vi "Begin(not).vi"(8 "error in":errorcluster) -> (0 "error out":errorcluster)   [LabVIEW 2016]
doc: "Called before other user functions, this VI is expected to open initial I/O refnums, load in file data, and do all program initialization. Notice that the <B>error out</B> terminal is simply used for data flow. Wiring it to other structures or subVIs ensures that this VI runs first."
uses:
  <vilib>/Rock Robotics/WPI/DriverStation/WPI_DriverStationRobotMode2.ctl
  <vilib>/Rock Robotics/WPI/Joystick/WPI_JoystickDeviceEnum.ctl
  <vilib>/Rock Robotics/WPI/ThirdParty/CanMotor/TalonSRX/WPI_CANTalonSRX_APIControlMode.ctl
  <vilib>/Rock Robotics/WPI/ThirdParty/CanMotor/TalonSRX/WPI_CANTalonSRX_APIFeedbackSelect.ctl
  <vilib>/Rock Robotics/SystemInterfaces/DIO/FPGA_DIOChannel.ctl
  <vilib>/Rock Robotics/SystemInterfaces/DIO/FPGA_DIOPWMChannel.ctl
  <vilib>/Rock Robotics/WPI/SafetyOutput/WPI_SafetyOutputConfigMenu.ctl
  Robot Global Data.vi
  <vilib>/Rock Robotics/Network Tables/NT Write String Array.vi
  <vilib>/Rock Robotics/WPI/Counter/WPI_CounterDigitalInputToDigitalSource.vi
  <vilib>/Rock Robotics/WPI/Switch/WPI_SwitchOpenLimit.vi
  <vilib>/Rock Robotics/WPI/RobotDrive/WPI_RobotDriveOpen4MotorWithExistingMotors.vi
  <vilib>/Rock Robotics/WPI/RobotDrive/WPI_RobotDriveOpen4MotorWithTalon.vi
  <vilib>/Rock Robotics/WPI/MotorControl/WPI_MotorControlOpen SPARK.vi
  <vilib>/Rock Robotics/WPI/MotorControl/WPI_MotorControlOpen Victor.vi
  <vilib>/Rock Robotics/WPI/Solenoid/WPI_SolenoidOpenSingle.vi
  <vilib>/Rock Robotics/WPI/Solenoid/WPI_SolenoidChannel.ctl
panel:
  in  "Number Encoder Lines\n(Counts Per Rotation)":u32=309
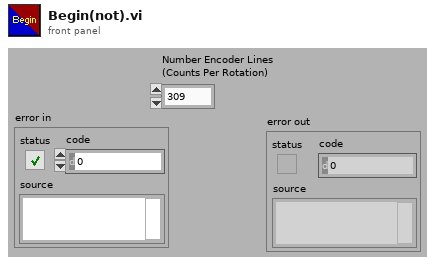
[diagram p1: front panel]
types:
  T1 = typedef "FPGA_DIOChannel.ctl" = enum8{"DIO 0", "DIO 1", "DIO 2", "DIO 3", "DIO 4", "DIO 5", "DIO 6", "DIO 7", "DIO 8", "DIO 9", "DIO MXP 0", "DIO MXP 1", "DIO MXP 2", "DIO MXP 3", "DIO MXP 4", "DIO MXP 5", "DIO MXP 6", "DIO MXP 7", "DIO MXP 8", "DIO MXP 9", "DIO MXP 10", "DIO MXP 11", "DIO MXP 12", "DIO MXP 13", "DIO MXP 14", "DIO MXP 15", "SPI Port CS1", "SPI Port CS2", "SPI Port CS3", "SPI Port MISO", "SPI Port MOSI", "Invalid"}
  T2 = typedef "WPI_CANTalonSRX_APIFeedbackSelect.ctl" = enum16{"Digital Quadrature Encoder", "Analog Potentiometer", "Analog Encoder", "Count on Quad-A (Rising-Edge)", "Count on Quad-A (Falling-Edge)", "CTR Magnetic Enc (Absolute)", "CTR Magnetic Enc (Relative)", "Pulse Width"}
  T3 = typedef "WPI_CANTalonSRX_APIControlMode.ctl" = enum8{"Percent VBus", "Speed", "Position", "Slave", "Unchanged / Invalid", "Voltage Compensation", "Current", "Motion Profile", "Motion Magic"}
  T4 = typedef "WPI_JoystickDeviceEnum.ctl" = enum16{"USB 0", "USB 1", "USB 2", "USB 3", "USB 4", "USB 5"}
  T5 = typedef "WPI_DriverStationRobotMode2.ctl" = enum16{"Autonomous Disabled", "Autonomous Enabled", "Teleop Disabled", "Teleop Enabled", "Disconnected", "Finish", "Test Disabled", "Test Enabled", "Emergency Stopped"}
  T6 = typedef "WPI_MotorControlDeviceRef.ctl" = cluster{"DeviceStatus":errorcluster, "Type":T7, "PWM":cluster{"PWM Channel":T8, "DeadBand":T9}, "CAN":cluster{"Device Number":u8, "SetOutput VI Ref":variant, "GetOutput VI Ref":variant, "Enable VI Ref":variant, "Disable VI Ref":variant, "Data":variant}, "Invert":bool}
  T7 = typedef "WPI_MotorControlType.ctl" = enum16{"PWM", "CAN"}
  T8 = typedef "FPGA_DIOPWMChannel.ctl" = enum8{"PWM 0", "PWM 1", "PWM 2", "PWM 3", "PWM 4", "PWM 5", "PWM 6", "PWM 7", "PWM 8", "PWM 9", "PWM MXP 0", "PWM MXP 1", "PWM MXP 2", "PWM MXP 3", "PWM MXP 4", "PWM MXP 5", "PWM MXP 6", "PWM MXP 7", "PWM MXP 8", "PWM MXP 9", "Invalid"}
  T9 = typedef "WPI_PWMDeadband.ctl" = cluster{"Name":string, "maxPositivePwm":i32, "minPositivePwm":i32, "centerPwm":i32, "maxNegativePwm":i32, "minNegativePwm":i32, "angularRange":u16}
  T10 = typedef "WPI_SafetyOutputConfigMenu.ctl" = enum16{"Enable", "Disable"}
  T11 = typedef "WPI_RobotDriveDevRef.ctl" = cluster{"DevStatus":errorcluster, "Motors[]":T6[], "Square Inputs":bool, "Max Output":dbl}
  T12 = typedef "WPI_ServoDeviceRef.ctl" = cluster{"DeviceStatus":errorcluster, "PWM Channel":T8, "DeadBand":T9}
  T13 = typedef "WPI_JoystickDevRef.ctl" = cluster{"Device":T4}
  T14 = typedef "WPI_SwitchDevRef.ctl" = cluster{"DevStatus":errorcluster, "DIO Channel":T1, "CntIndex":T15, "Normally Closed":bool}
  T15 = typedef "FPGA_CounterCtrSystemIndex.ctl" = enum8{"Ctr 0", "Ctr 1", "Ctr 2", "Ctr 3", "Ctr 4", "Ctr 5", "Ctr 6", "Ctr 7", "Invalid"}
  T16 = typedef "WPI_SolenoidChannel.ctl" = enum8{"Solenoid 0", "Solenoid 1", "Solenoid 2", "Solenoid 3", "Solenoid 4", "Solenoid 5", "Solenoid 6", "Solenoid 7", "Invalid"}
  T17 = typedef "WPI_SolenoidDevRef.ctl" = cluster{"DevStatus":errorcluster, "Pneumatics Control Module":u8, "Forward Solenoid Channel":T16, "Reverse Solenoid Channel":T16}
  T18 = typedef "WPI_DigitalInputDevRef.ctl" = cluster{"DevStatus":errorcluster, "DIO Channel":T1}
  T19 = typedef "FPGA_CounterEncoderSourceConvertionLVSourceType.ctl" = cluster{"DevStatus":errorcluster, "AnalogTriggerMode?":bool, "DigitalMode":cluster{"DIO Channel":T20}, "AnalogTriggerMode":cluster{"AnalogTriggerIndex":T21, "OutputType":T22}}
  T20 = typedef "FPGA_DIODigitalSourceChannel.ctl" = enum8{"DIO 0", "DIO 1", "DIO 2", "DIO 3", "DIO 4", "DIO 5", "DIO 6", "DIO 7", "DIO 8", "DIO 9", "DIO MXP 0", "DIO MXP 1", "DIO MXP 2", "DIO MXP 3", "DIO MXP 4", "DIO MXP 5", "DIO MXP 6", "DIO MXP 7", "DIO MXP 8", "DIO MXP 9", "DIO MXP 10", "DIO MXP 11", "DIO MXP 12", "DIO MXP 13", "DIO MXP 14", "DIO MXP 15", "Disabled"}
  T21 = typedef "FPGA_AnalogTriggerIndex.ctl" = enum8{"Trig 0", "Trig 1", "Trig 2", "Trig 3", "Trig 4", "Trig 5", "Trig 6", "Trig 7", "Invalid"}
  T22 = typedef "FPGA_AnalogTriggerOutType.ctl" = enum16{"InWindow", "TriggerState", "Rising", "Falling"}
  T23 = typedef "WPI_EncoderDevRef.ctl" = cluster{"DevStatus":errorcluster, "EncoderIndex":T24, "CounterIndex":T15, "DistancePerCount":dbl, "Decoding Type":T25}
  T24 = typedef "FPGA_EncoderIdx.ctl" = enum8{"Enc 0", "Enc 1", "Enc 2", "Enc 3", "Enc 4", "Enc 5", "Enc 6", "Enc 7", "Invalid"}
  T25 = typedef "WPI_EncoderType.ctl" = enum16{"1x", "2x", "4x"}
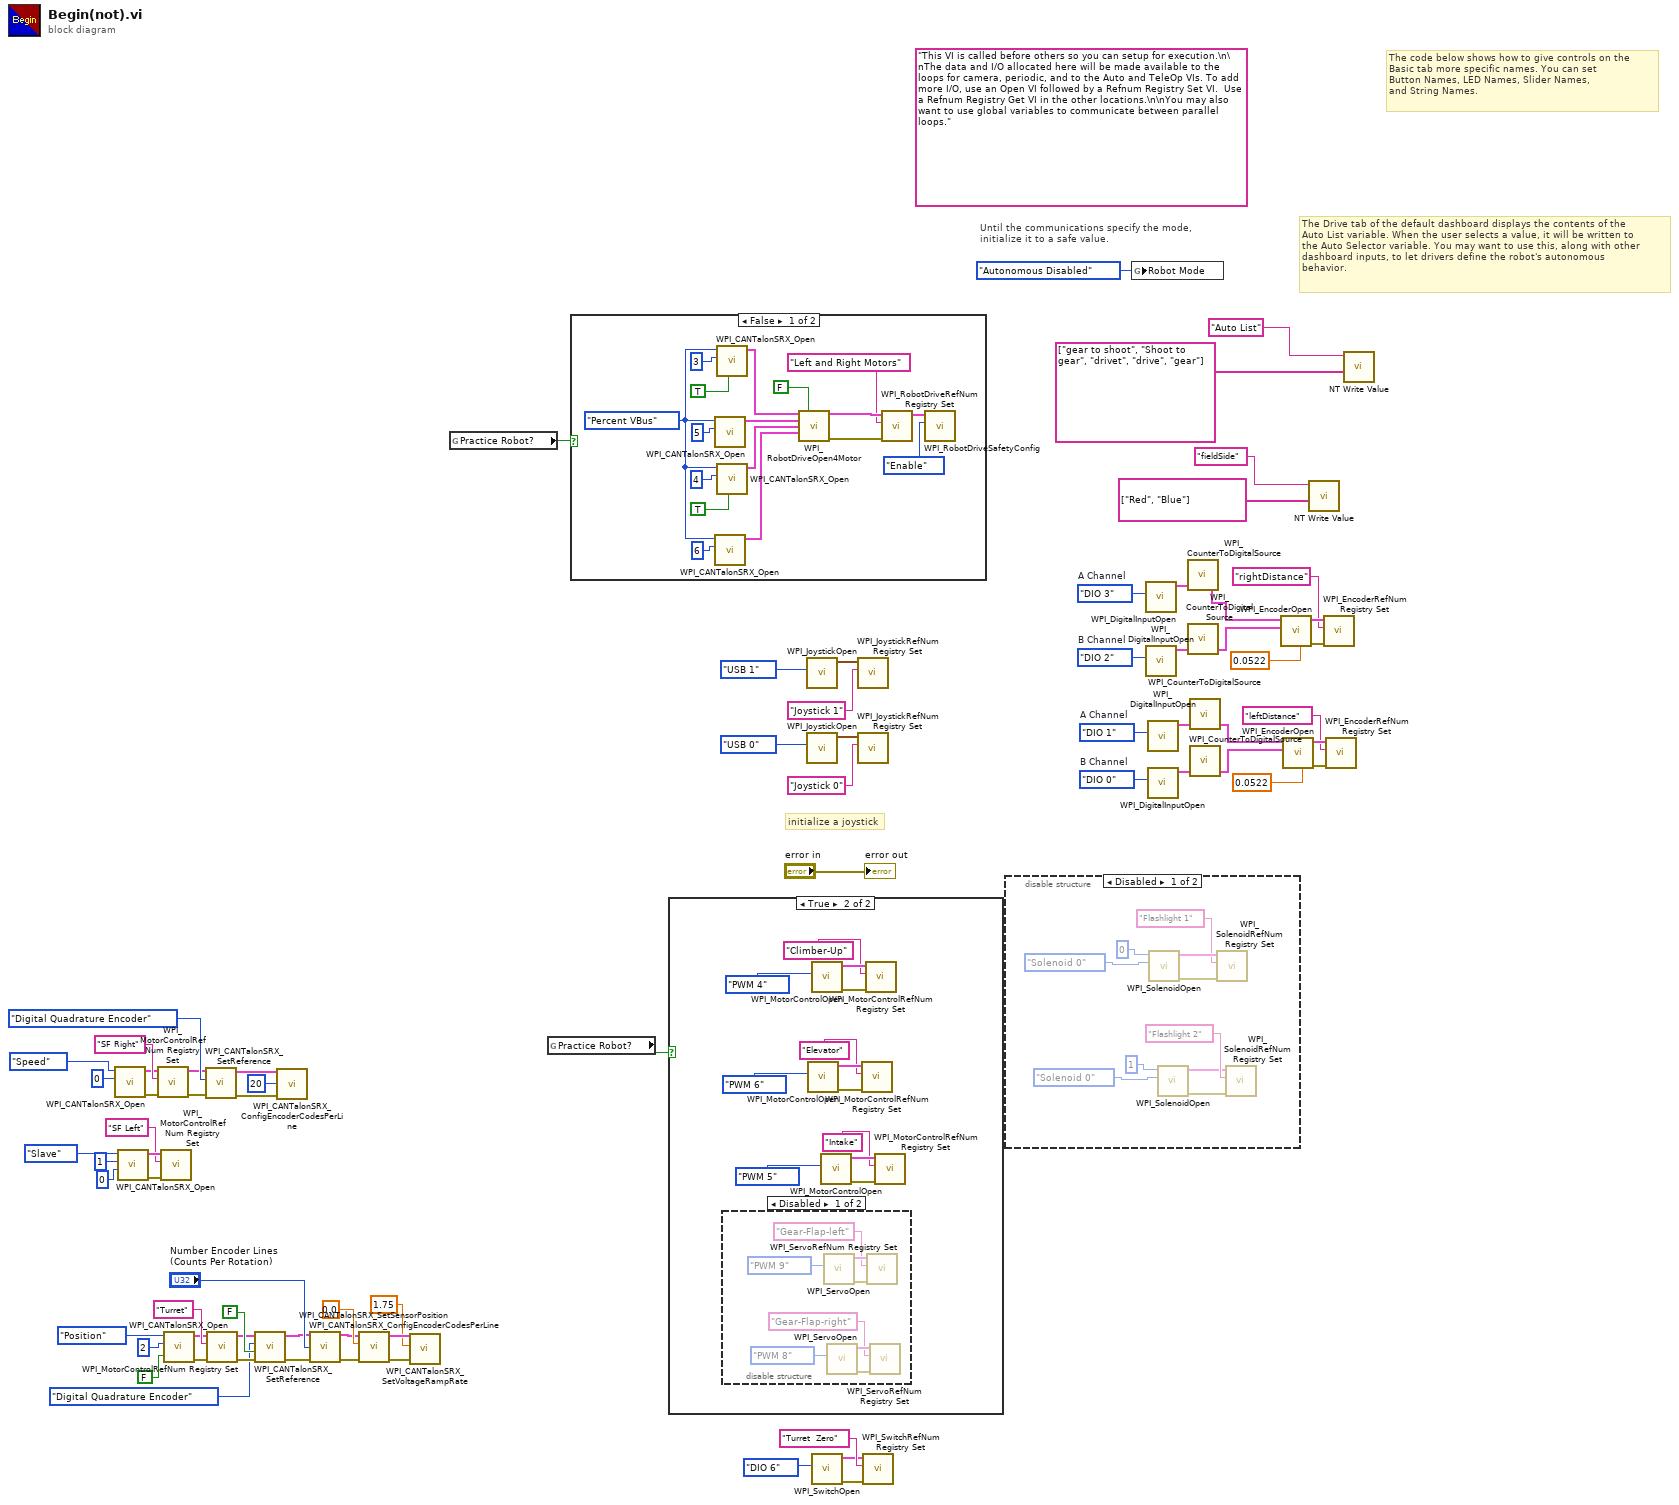
[diagram p0: block diagram]
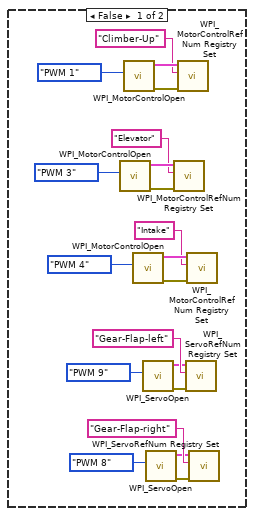
[diagram p3: hidden frame]
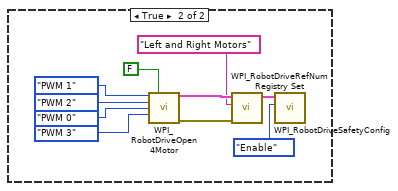
[diagram p5: hidden frame]
diagram:
  w18 = FPGA_DIOChannel."DIO 2"  # B Channel
  w17 = FPGA_DIOChannel."DIO 3"  # A Channel
  w27 = FPGA_DIOChannel."DIO 0"  # B Channel
  w26 = FPGA_DIOChannel."DIO 1"  # A Channel
  (unwired) "This VI is called before others so you can setup for execution.\n\nThe data and I/O allocated here will be made available to the loops for camera, periodic, and to the Auto and TeleOp VIs. To add more I/O, use an Open VI followed by a Refnum Registry Set VI.  Use a Refnum Registry Get VI in the other locations.\n\nYou may also want to use global variables to communicate between parallel loops."
  # "The Drive tab of the default dashboard displays the contents of the\nAuto List variable. When the user selects a value, it will be written to\nthe Auto Selector variable. You may want to use this, along with other\ndashboard inputs, to let drivers define the robot's autonomous\nbehavior."
  # "The code below shows how to give controls on the\nBasic tab more specific names. You can set\nButton Names, LED Names, Slider Names,\nand String Names."
  # "initialize a joystick"
  # "Until the communications specify the mode,\ninitialize it to a safe value."
  n1 = call <vilib>:"WPI_CANTalonSRX_Open.vi"("Device Number"=u8 0, "Control Mode"=WPI_CANTalonSRX_APIControlMode."Speed") -> ("error out"=w48:errorcluster, "CAN Talon SRX Ref"=w47:T6)  [unwired: 8 in]
  n2 = call <vilib>:"WPI_CANTalonSRX_Open.vi"("Master Device Number"=u8 0, "Device Number"=u8 1, "Control Mode"=WPI_CANTalonSRX_APIControlMode."Slave") -> ("error out"=w55:errorcluster, "CAN Talon SRX Ref"=w56:T6)  [unwired: 7 in]
  n3 = call <vilib>:"WPI_MotorControlRefNum Registry Set.vi"("error in (no error)"=w48, "refnum name"="SF Right", "MotorControlDevRef"=w47) -> ("error out"=w29:errorcluster, "MotorControlDevRef"=w30:T6)  [unwired: 7 in]
  n4 = call <vilib>:"WPI_MotorControlRefNum Registry Set.vi"("error in (no error)"=w55, "refnum name"="SF Left", "MotorControlDevRef"=w56) -> ()  [unwired: 7 in, 2 out]
  n5 = call <vilib>:"WPI_CANTalonSRX_Open.vi"("Invert"=FALSE, "Device Number"=u8 2, "Control Mode"=WPI_CANTalonSRX_APIControlMode."Position") -> ("error out"=w39:errorcluster, "CAN Talon SRX Ref"=w41:T6)  [unwired: 7 in]
  n6 = call <vilib>:"WPI_CANTalonSRX_SetReference.vi"("error in (no error)"=w29, "Feedback Reference"=WPI_CANTalonSRX_APIFeedbackSelect."Digital Quadrature Encoder", "CAN Talon SRX Ref"=w30) -> ("error out"=w28:errorcluster, "CAN Talon SRX Ref"=w33:T6)  [unwired: 7 in]
  n7 = call <vilib>:"WPI_MotorControlRefNum Registry Set.vi"("error in (no error)"=w39, "refnum name"="Turret", "MotorControlDevRef"=w41) -> ("error out"=w38:errorcluster, "MotorControlDevRef"=w40:T6)  [unwired: 7 in]
  n8 = call <vilib>:"WPI_CANTalonSRX_SetReference.vi"("error in (no error)"=w38, "Reverse Feedback Sensor"=FALSE, "Feedback Reference"=WPI_CANTalonSRX_APIFeedbackSelect."Digital Quadrature Encoder", "CAN Talon SRX Ref"=w40) -> ("error out"=w37:errorcluster, "CAN Talon SRX Ref"=w43:T6)  [unwired: 6 in]
  n9 = call <vilib>:"WPI_CANTalonSRX_ConfigEncoderCodesPerLine.vi"("CAN Talon SRX Ref"=w33, "Number Encoder Lines\n(Counts Per Rotation)"=u32 20 ("Number Encoder Lines\n(Counts Per Rotation)"), "error in (no error)"=w28) -> ()  [unwired: 11 in, 2 out]
  n10 = call <vilib>:"WPI_CANTalonSRX_ConfigEncoderCodesPerLine.vi"("CAN Talon SRX Ref"=w43, "Number Encoder Lines\n(Counts Per Rotation)"="Number Encoder Lines\n(Counts Per Rotation)", "error in (no error)"=w37) -> ("CAN Talon SRX Ref"=w35:T6, "error out"=w36:errorcluster)  [unwired: 11 in]
  n11 = call <vilib>:"WPI_CANTalonSRX_SetSensorPosition.vi"("error in (no error)"=w36, "New Sensor Position"=0.0, "CAN Talon SRX Ref"=w35) -> ("error out"=w3:errorcluster, "CAN Talon SRX Ref"=w2:T6)  [unwired: 7 in]
  n12 = call <vilib>:"WPI_CANTalonSRX_SetVoltageRampRate.vi"("error in (no error)"=w3, "Throttle Ramp Rate (percent/s)"=1.75, "CAN Talon SRX Ref"=w2) -> ()  [unwired: 7 in, 2 out]
  n13 = global read "Robot Global Data.vi" "Practice Robot?"() -> (w62:bool)
  n14 = global read "Robot Global Data.vi" "Practice Robot?"() -> (w61:bool)
  n15 = case shown="False" w62 {
    frame False {
      w82 = WPI_CANTalonSRX_APIControlMode."Percent VBus" ("Control Mode")
      n16 = call <vilib>:"WPI_CANTalonSRX_Open.vi"("Device Number"=u8 5, "Control Mode"=w82) -> ("CAN Talon SRX Ref"=w85:T6)  [unwired: 8 in, 1 out]
      n17 = call <vilib>:"WPI_CANTalonSRX_Open.vi"("Device Number"=u8 6, "Control Mode"=w82) -> ("CAN Talon SRX Ref"=w83:T6)  [unwired: 8 in, 1 out]
      n18 = call <vilib>:"WPI_CANTalonSRX_Open.vi"("Invert"=TRUE, "Device Number"=u8 3, "Control Mode"=w82) -> ("CAN Talon SRX Ref"=w86:T6)  [unwired: 7 in, 1 out]
      n19 = call <vilib>:"WPI_CANTalonSRX_Open.vi"("Invert"=TRUE, "Device Number"=u8 4, "Control Mode"=w82) -> ("CAN Talon SRX Ref"=w84:T6)  [unwired: 7 in, 1 out]
      n20 = call-poly <vilib>:"WPI_RobotDriveOpen4Motor.vi"("Rear Left Motor Dev Ref"=w86, "Square Inputs"=FALSE, "Rear Right Motor Dev Ref"=w85, "Front Left Motor Dev Ref"=w84, "Front Right Motor Dev Ref"=w83) -> ("RobotDriveDevRef"=w91:T11, "error out"=w89:errorcluster)  [unwired: 9 in]
      n21 = call <vilib>:"WPI_RobotDriveRefNum Registry Set.vi"("error in (no error)"=w89, "refnum name"="Left and Right Motors", "RobotDriveDevRef"=w91) -> ("RobotDriveDevRef"=w88:T11)  [unwired: 1 in, 7 out]
      n22 = call <vilib>:"WPI_RobotDriveSafetyConfig.vi"("mode"=WPI_SafetyOutputConfigMenu."Enable", "RobotDriveDevRef"=w88) -> ()  [unwired: 8 in, 2 out]
    }
    frame True {
      n23 = call-poly <vilib>:"WPI_RobotDriveOpen4Motor.vi"("Rear Left Motor"=FPGA_DIOPWMChannel."PWM 1", "Rear Left Motor Inverted"=FALSE ("Square Inputs"), "Rear Right Motor"=FPGA_DIOPWMChannel."PWM 2", "Front Left Motor"=FPGA_DIOPWMChannel."PWM 0", "Front Right Motor"=FPGA_DIOPWMChannel."PWM 3") -> ("RobotDriveDevRef"=w101:T11, "error out"=w99:errorcluster)  [unwired: 9 in]
      n24 = call <vilib>:"WPI_RobotDriveRefNum Registry Set.vi"("error in (no error)"=w99, "refnum name"="Left and Right Motors", "RobotDriveDevRef"=w101) -> ("RobotDriveDevRef"=w98:T11)  [unwired: 1 in, 7 out]
      n25 = call <vilib>:"WPI_RobotDriveSafetyConfig.vi"("mode"=WPI_SafetyOutputConfigMenu."Enable", "RobotDriveDevRef"=w98) -> ()  [unwired: 8 in, 2 out]
    }
  }
  n26 = case shown="True" w61 {
    frame False {
      n27 = call-poly <vilib>:"WPI_MotorControlOpen.vi"("PWM Channel"=FPGA_DIOPWMChannel."PWM 3") -> ("error out"=w121:errorcluster, "MotorControlDeviceRef"=w120:T6)  [unwired: 9 in]
      n28 = call-poly <vilib>:"WPI_MotorControlOpen.vi"("PWM Channel"=FPGA_DIOPWMChannel."PWM 1") -> ("error out"=w117:errorcluster, "MotorControlDeviceRef"=w116:T6)  [unwired: 9 in]
      n29 = call-poly <vilib>:"WPI_MotorControlOpen.vi"("PWM Channel"=FPGA_DIOPWMChannel."PWM 4") -> ("error out"=w113:errorcluster, "MotorControlDeviceRef"=w112:T6)  [unwired: 9 in]
      n30 = call <vilib>:"WPI_ServoOpen.vi"("PWM Channel"=FPGA_DIOPWMChannel."PWM 9") -> ("error out"=w107:errorcluster, "ServoDeviceRef"=w102:T12)  [unwired: 9 in]
      n31 = call <vilib>:"WPI_ServoOpen.vi"("PWM Channel"=FPGA_DIOPWMChannel."PWM 8") -> ("error out"=w106:errorcluster, "ServoDeviceRef"=w103:T12)  [unwired: 9 in]
      n32 = call <vilib>:"WPI_MotorControlRefNum Registry Set.vi"("error in (no error)"=w121, "refnum name"="Elevator", "MotorControlDevRef"=w120) -> ()  [unwired: 7 in, 2 out]
      n33 = call <vilib>:"WPI_MotorControlRefNum Registry Set.vi"("error in (no error)"=w117, "refnum name"="Climber-Up", "MotorControlDevRef"=w116) -> ()  [unwired: 7 in, 2 out]
      n34 = call <vilib>:"WPI_ServoRefNum Registry Set.vi"("error in (no error)"=w107, "refnum name"="Gear-Flap-left", "ServoDeviceRef"=w102) -> ()  [unwired: 7 in, 2 out]
      n35 = call <vilib>:"WPI_MotorControlRefNum Registry Set.vi"("error in (no error)"=w113, "refnum name"="Intake", "MotorControlDevRef"=w112) -> ()  [unwired: 7 in, 2 out]
      n36 = call <vilib>:"WPI_ServoRefNum Registry Set.vi"("error in (no error)"=w106, "refnum name"="Gear-Flap-right", "ServoDeviceRef"=w103) -> ()  [unwired: 7 in, 2 out]
    }
    frame True {
      n37 = disable-structure shown="Disabled" {
        frame Disabled {
          n38 = call <vilib>:"WPI_ServoOpen.vi"("PWM Channel"=FPGA_DIOPWMChannel."PWM 9") -> ("error out"=w136:errorcluster, "ServoDeviceRef"=w141:T12)  [unwired: 9 in]
          n39 = call <vilib>:"WPI_ServoOpen.vi"("PWM Channel"=FPGA_DIOPWMChannel."PWM 8") -> ("error out"=w137:errorcluster, "ServoDeviceRef"=w140:T12)  [unwired: 9 in]
          n40 = call <vilib>:"WPI_ServoRefNum Registry Set.vi"("error in (no error)"=w136, "refnum name"="Gear-Flap-left", "ServoDeviceRef"=w141) -> ()  [unwired: 7 in, 2 out]
          n41 = call <vilib>:"WPI_ServoRefNum Registry Set.vi"("error in (no error)"=w137, "refnum name"="Gear-Flap-right", "ServoDeviceRef"=w140) -> ()  [unwired: 7 in, 2 out]
        }
        frame Enabled {
        }
      }
      n42 = call-poly <vilib>:"WPI_MotorControlOpen.vi"("PWM Channel"=FPGA_DIOPWMChannel."PWM 6") -> ("error out"=w133:errorcluster, "MotorControlDeviceRef"=w132:T6)  [unwired: 9 in]
      n43 = call-poly <vilib>:"WPI_MotorControlOpen.vi"("PWM Channel"=FPGA_DIOPWMChannel."PWM 4") -> ("error out"=w129:errorcluster, "MotorControlDeviceRef"=w128:T6)  [unwired: 9 in]
      n44 = call-poly <vilib>:"WPI_MotorControlOpen.vi"("PWM Channel"=FPGA_DIOPWMChannel."PWM 5") -> ("error out"=w125:errorcluster, "MotorControlDeviceRef"=w124:T6)  [unwired: 9 in]
      n45 = call <vilib>:"WPI_MotorControlRefNum Registry Set.vi"("error in (no error)"=w133, "refnum name"="Elevator", "MotorControlDevRef"=w132) -> ()  [unwired: 7 in, 2 out]
      n46 = call <vilib>:"WPI_MotorControlRefNum Registry Set.vi"("error in (no error)"=w129, "refnum name"="Climber-Up", "MotorControlDevRef"=w128) -> ()  [unwired: 7 in, 2 out]
      n47 = call <vilib>:"WPI_MotorControlRefNum Registry Set.vi"("error in (no error)"=w125, "refnum name"="Intake", "MotorControlDevRef"=w124) -> ()  [unwired: 7 in, 2 out]
    }
  }
  n48 = call <vilib>:"WPI_JoystickOpen.vi"("JoystickDevice"=WPI_JoystickDeviceEnum."USB 1") -> ("JoystickDevRef"=w65:T13)  [unwired: 10 in]
  n49 = call <vilib>:"WPI_JoystickOpen.vi"("JoystickDevice"=WPI_JoystickDeviceEnum."USB 0") -> ("JoystickDevRef"=w72:T13)  [unwired: 10 in]
  n50 = call-poly <vilib>:"WPI_SwitchOpen.vi"("DIO Channel"=FPGA_DIOChannel."DIO 6") -> ("error out"=w5:errorcluster, "SwitchDevRef"=w6:T14)  [unwired: 9 in]
  n51 = call <vilib>:"WPI_JoystickRefNum Registry Set.vi"("refnum name"="Joystick 1", "JoystickDevRef"=w65) -> ()  [unwired: 8 in, 2 out]
  n52 = call <vilib>:"WPI_JoystickRefNum Registry Set.vi"("refnum name"="Joystick 0", "JoystickDevRef"=w72) -> ()  [unwired: 8 in, 2 out]
  n53 = call <vilib>:"WPI_SwitchRefNum Registry Set.vi"("error in (no error)"=w5, "refnum name"="Turret  Zero", "SwitchDevRef"=w6) -> ()  [unwired: 7 in, 2 out]
  n54 = disable-structure shown="Disabled" {
    frame Disabled {
      n55 = call-poly <vilib>:"WPI_SolenoidOpen.vi"("Solenoid Channel"=WPI_SolenoidChannel."Solenoid 0", "Pneumatics Control Module (0)"=u8 0) -> ("error out"=w149:errorcluster, "SolenoidDevRef"=w148:T17)  [unwired: 8 in]
      n56 = call-poly <vilib>:"WPI_SolenoidOpen.vi"("Solenoid Channel"=WPI_SolenoidChannel."Solenoid 0", "Pneumatics Control Module (0)"=u8 1) -> ("error out"=w144:errorcluster, "SolenoidDevRef"=w145:T17)  [unwired: 8 in]
      n57 = call <vilib>:"WPI_SolenoidRefNum Registry Set.vi"("error in (no error)"=w149, "refnum name"="Flashlight 1", "SolenoidDevRef"=w148) -> ()  [unwired: 7 in, 2 out]
      n58 = call <vilib>:"WPI_SolenoidRefNum Registry Set.vi"("error in (no error)"=w144, "refnum name"="Flashlight 2", "SolenoidDevRef"=w145) -> ()  [unwired: 7 in, 2 out]
    }
    frame Enabled {
    }
  }
  n59 = global write "Robot Global Data.vi" "Robot Mode"(WPI_DriverStationRobotMode2."Autonomous Disabled" ("Robot Mode")) -> ()
  n60 = call <vilib>:"WPI_DigitalInputOpen.vi"("DIO Channel"=w17) -> ("DigitalInputDevRef"=w14:T18)  [unwired: 1 in, 9 out]
  n61 = call <vilib>:"WPI_DigitalInputOpen.vi"("DIO Channel"=w18) -> ("DigitalInputDevRef"=w15:T18)  [unwired: 1 in, 9 out]
  n62 = call <vilib>:"WPI_DigitalInputOpen.vi"("DIO Channel"=w26) -> ("DigitalInputDevRef"=w23:T18)  [unwired: 1 in, 9 out]
  n63 = call <vilib>:"WPI_DigitalInputOpen.vi"("DIO Channel"=w27) -> ("DigitalInputDevRef"=w24:T18)  [unwired: 1 in, 9 out]
  n64 = call-poly <vilib>:"WPI_CounterToDigitalSource.vi"("DigitalInputDevRef"=w14) -> ("Digital Source"=w13:T19)  [unwired: 6 out]
  n65 = call-poly <vilib>:"WPI_CounterToDigitalSource.vi"("DigitalInputDevRef"=w15) -> ("Digital Source"=w16:T19)  [unwired: 6 out]
  n66 = call-poly <vilib>:"WPI_CounterToDigitalSource.vi"("DigitalInputDevRef"=w23) -> ("Digital Source"=w22:T19)  [unwired: 6 out]
  n67 = call-poly <vilib>:"WPI_CounterToDigitalSource.vi"("DigitalInputDevRef"=w24) -> ("Digital Source"=w25:T19)  [unwired: 6 out]
  n68 = call <vilib>:"WPI_EncoderOpen.vi"("DistancePerCount"=0.0522, "BSource"=w16, "ASource"=w13) -> ("error out"=w12:errorcluster, "EncoderDevRef"=w11:T23)  [unwired: 5 in, 2 out]
  n69 = call <vilib>:"WPI_EncoderOpen.vi"("DistancePerCount"=0.0522, "BSource"=w25, "ASource"=w22) -> ("error out"=w21:errorcluster, "EncoderDevRef"=w20:T23)  [unwired: 5 in, 2 out]
  n70 = call-poly <vilib>:"NT Write Value.vi"("String Array"=string[] ["Red", "Blue"], "Name"="fieldSide") -> ()  [unwired: 9 in, 1 out]
  n71 = call <vilib>:"WPI_EncoderRefNum Registry Set.vi"("error in (no error)"=w12, "refnum name"="rightDistance", "EncoderDevRef"=w11) -> ()  [unwired: 7 in, 2 out]
  n72 = call <vilib>:"WPI_EncoderRefNum Registry Set.vi"("error in (no error)"=w21, "refnum name"="leftDistance", "EncoderDevRef"=w20) -> ()  [unwired: 7 in, 2 out]
  n73 = call-poly <vilib>:"NT Write Value.vi"("String Array"=string[] ["gear to shoot", "Shoot to gear", "drivet", "drive", "gear"], "Name"="Auto List") -> ()  [unwired: 9 in, 1 out]
  "error out" <- "error in"
